vi "average-20220125.vi"(9 "3":dbl[](array[numeric]), 10 "2":dbl[](array[numeric]), 11 "1":dbl[](array[numeric])) -> (0 "Array":dbl[](array[numeric]), 1 "element 3":dbl, 2 "element 2":dbl, 3 "element":dbl)   [LabVIEW 2019]
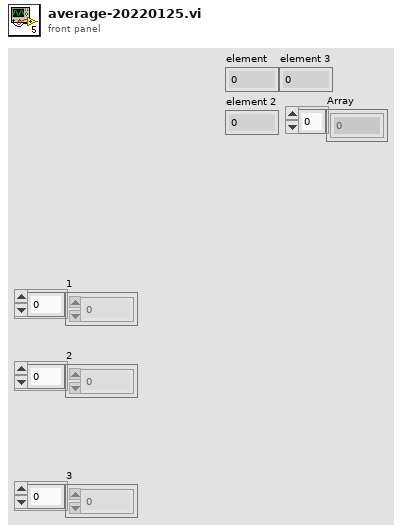
[diagram p1: front panel]
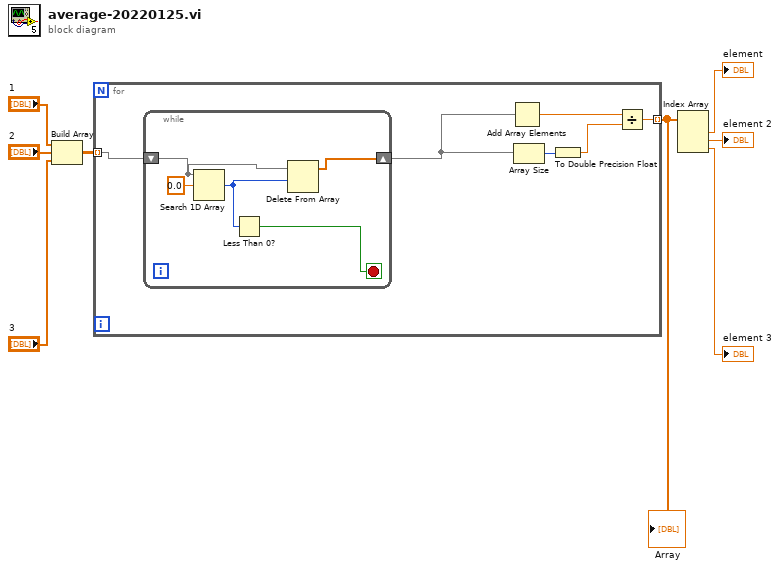
[diagram p0: block diagram]
diagram:
  n1 = Build Array("1", "2", "3") -> (w5:dbl[][])
  n2 = for {
    tunnel: w5 -> [w10] mode=indexing
    tunnel: [w12] -> w4 mode=indexing
    n3 = while {
      shift-right: [w15] -> w9
      shift-left: w10 -> [w18]
      stop <- w16 stop-if-true
      n4 = Search 1D Array(1D array=w18, element=0.0) -> (index of element=w17:i32)  [unwired: 1 in]
      n5 = Less Than 0?(x=w17) -> (x < 0?=w16:bool)
      n6 = Delete From Array(array=w18, length=w17) -> (array with subset deleted=w15:dbl[])  [unwired: 1 in, 1 out]
    }
    n7 = Add Array Elements(numeric array=w9) -> (sum=w14:dbl)
    n8 = Array Size(array=w9) -> (size(s)=w13:i32)
    n9 = To Double Precision Float(number=w13) -> (double precision float=w11:dbl)
    n10 = Divide(x=w14, y=w11) -> (x/y=w12:dbl)
  }
  "Array" <- w4
  n11 = Index Array(array=w4) -> (element #1=→"element":dbl, element #2=→"element 2":dbl, element #3=→"element 3":dbl)  [unwired: 3 in]
